vi "ScriptParser.vi"(0 "File Path Control":path, 1 "storage refnum (file) out":refnum<k20>, 2 "ResultaFileName":string, 3 "Array":string[](array[string]), 4 "I":dbl) -> ()   [LabVIEW 2014]
uses:
  <vilib>/Platform/storage/Storage.llb/usiSequenceRepresentation.ctl
  <vilib>/Platform/storage/lvStorage.llb/_queryPropPoly.vi
  <vilib>/Platform/storage/lvStorage.llb/_queryPropString.vi
  <vilib>/Platform/storage/lvStorage.llb/_queryGenericObjects.vi
  <vilib>/Platform/storage/lvStorage.llb/_loadAllDdt.vi
  <vilib>/Platform/storage/lvStorage.llb/xStorage/xStorageSupp/ErrorOut.vi
  <vilib>/Platform/storage/lvStorage.llb/_createOrGetByNameExplicitChildObject.vi
  <vilib>/Platform/storage/Storage.llb/__savePropString.vi
  <vilib>/Platform/storage/lvStorage.llb/__saveFloat64Channel.vi
  <vilib>/Platform/storage/lvStorage.llb/_openStorageWithRootAutoDetect.vi
  <vilib>/Platform/storage/Storage.llb/__savePropTime.vi
  <vilib>/Platform/storage/Storage.llb/Get Object Info.vi
  <vilib>/Platform/storage/Storage.llb/__closeStorageFromObject.vi
  <vilib>/Platform/storage/lvStorage.llb/xStorage/Read Data/Read Data.xnode
  <vilib>/Platform/storage/lvStorage.llb/xStorage/Write Data/Write Data.xnode
  <vilib>/Platform/storage/lvStorage.llb/xStorage/Open Data Storage/Open Data Storage.xnode
  <vilib>/Platform/storage/lvStorage.llb/xStorage/Set Properties/Set Properties.xnode
  <vilib>/Platform/storage/lvStorage.llb/xStorage/Close Data Storage/Close Data Storage.xnode
panel:
  out "Numeric":dbl
  out "storage refnums (channel)":refnum<k20>[](array[refnum])
  out "Default":bool
  # "DEBUG"
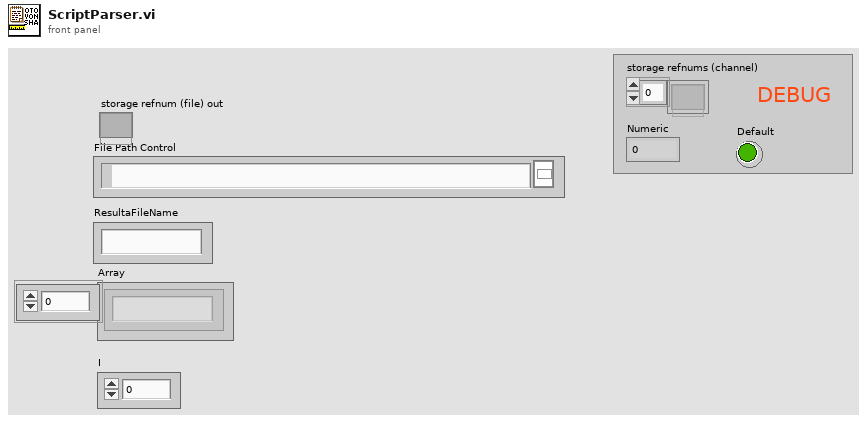
[diagram p1: front panel]
types:
  T1 = enum16{"UPDATE", "READ", "QUERY", "CREATE CHILD", "CREATE", "CONNECT", "DISCONNECT"}
  T2 = enum16{"Append values", "Replace values at index", "Replace all values"}
  T3 = typedef "usiSequenceRepresentation.ctl" = enum16{"explicit", "implicit"}
  T4 = enum16{"open", "open or create", "create or replace", "create", "open (read only)"}
  T5 = typedef "Channel.ctl" = cluster{"AutoLevel":bool, "Thresold":dbl, "Impedance ":dbl, "Voltage Range":dbl, "Active Edge ":i32}
  T6 = typedef "VBreakInitialCond.ctl" = cluster{"Range":dbl, "Ilim":dbl, "Level":dbl, "Channel":i32, "Timed Totalize":dbl}
  T7 = typedef "VBreakStopCondition.ctl" = cluster{"Count Min":dbl, "Count Max":dbl, "Vmax":dbl}
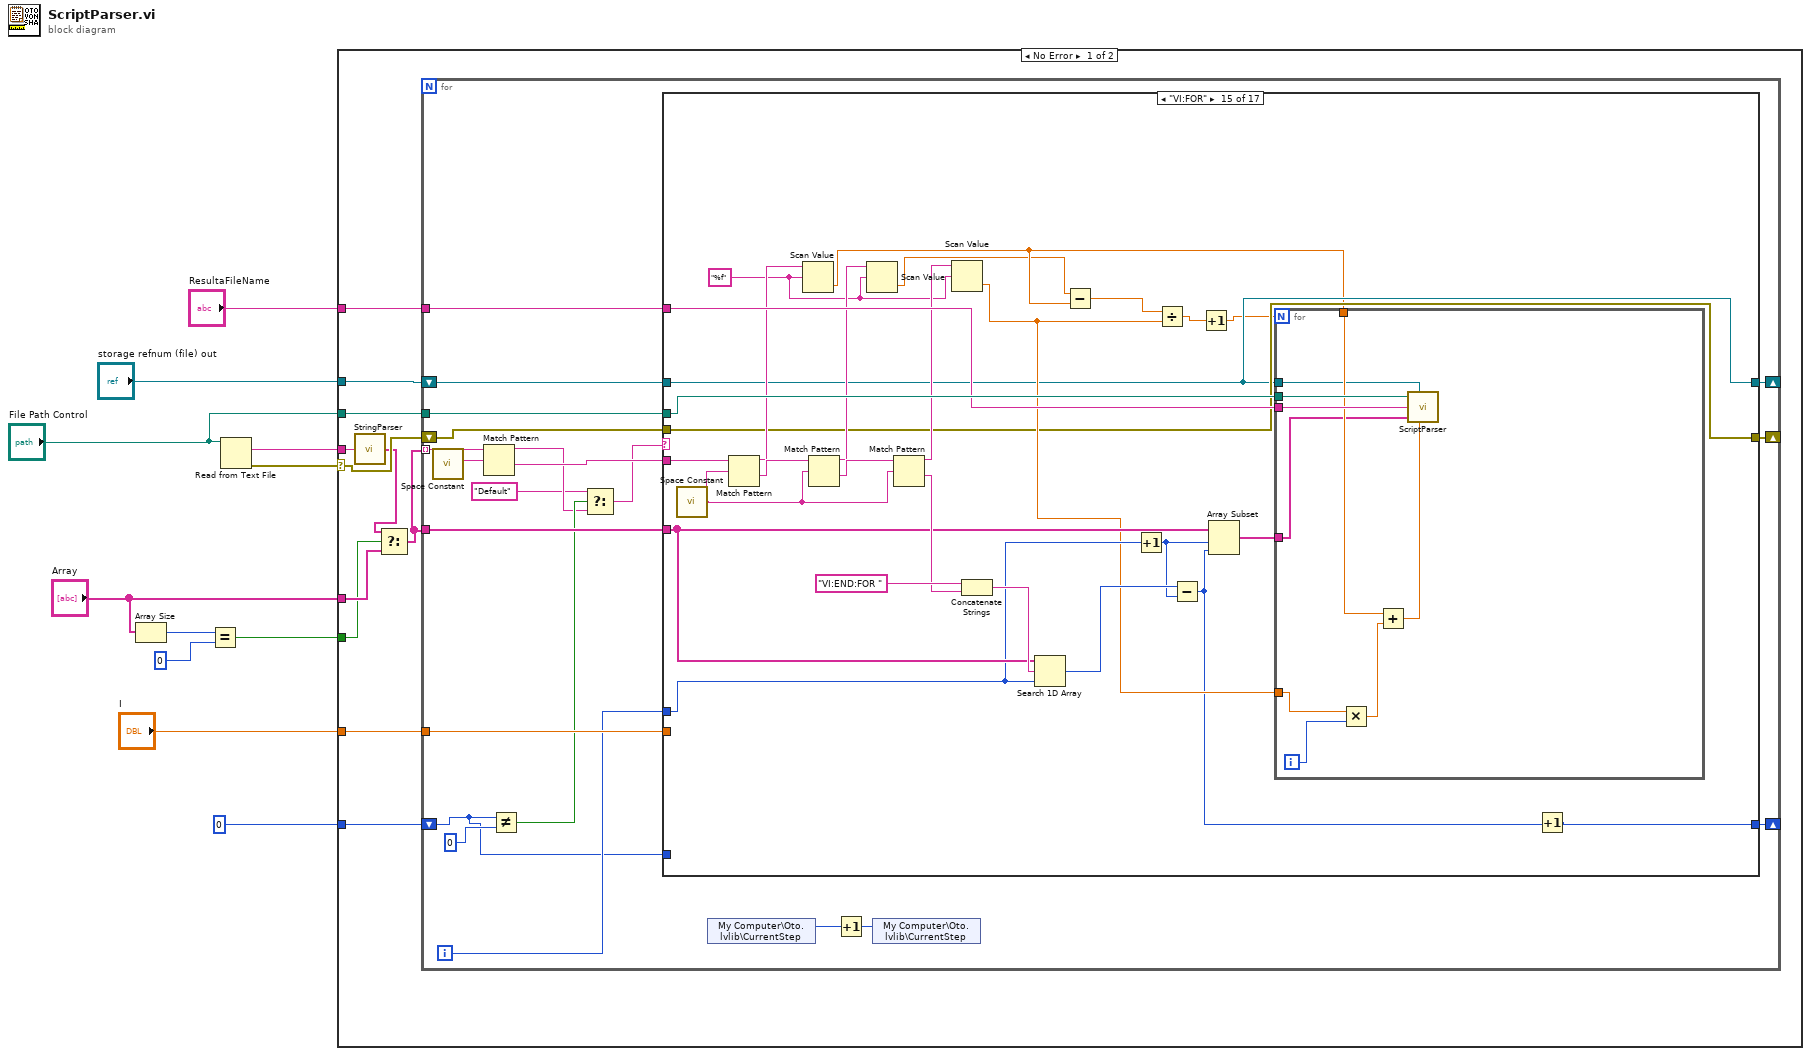
[diagram p0: block diagram]
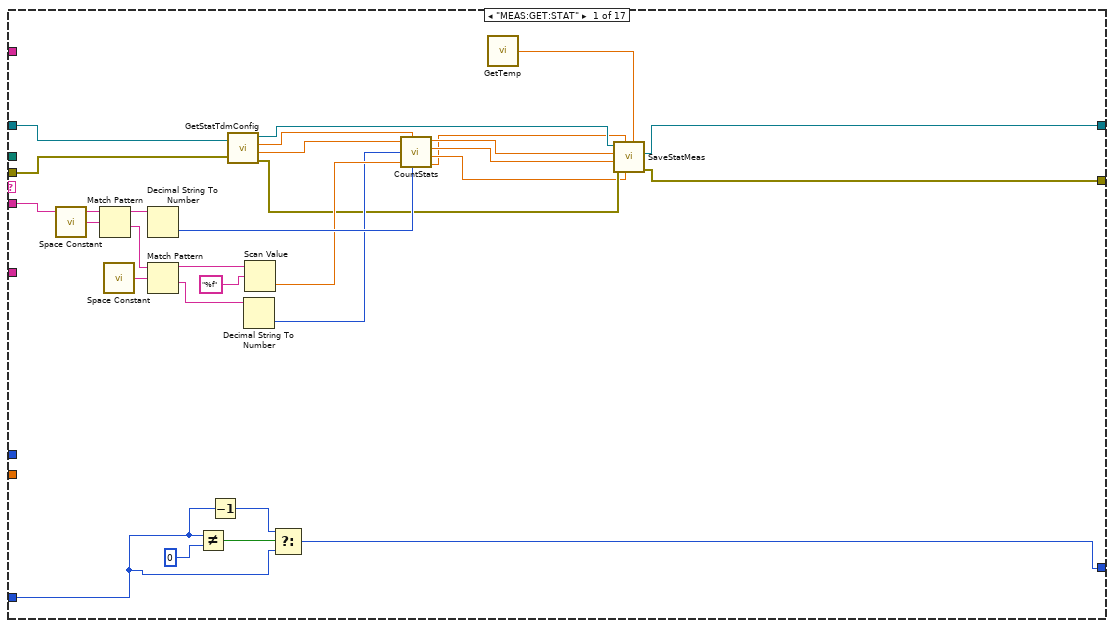
[diagram p2: hidden frame]
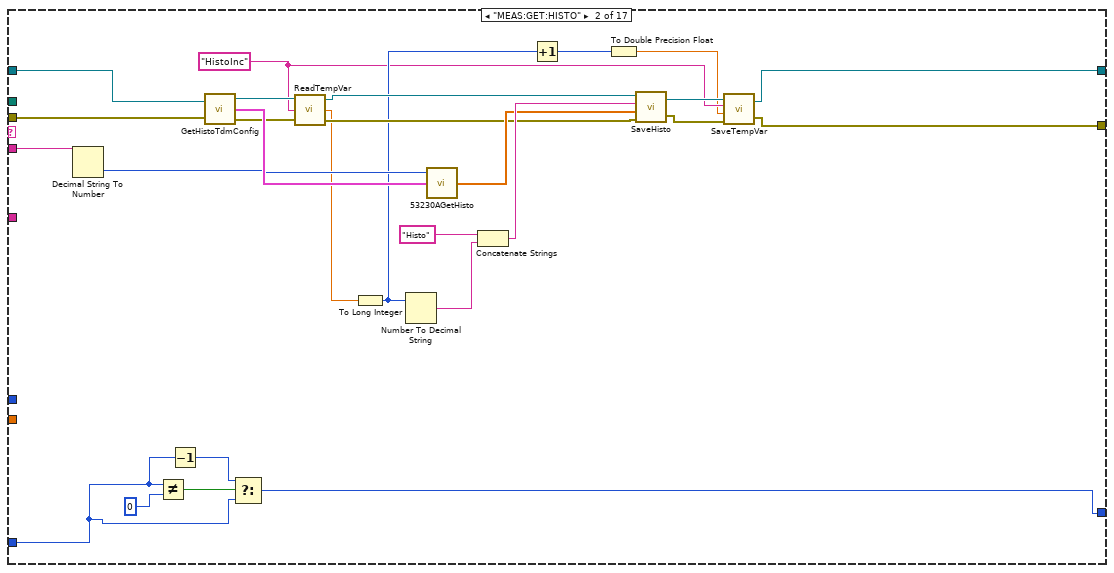
[diagram p3: hidden frame]
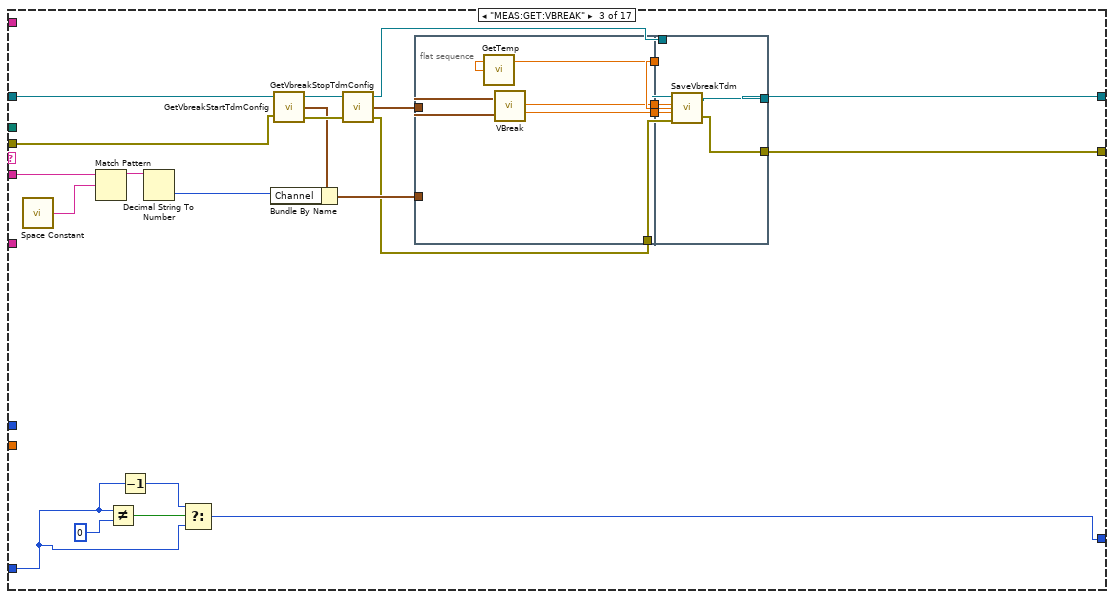
[diagram p4: hidden frame]
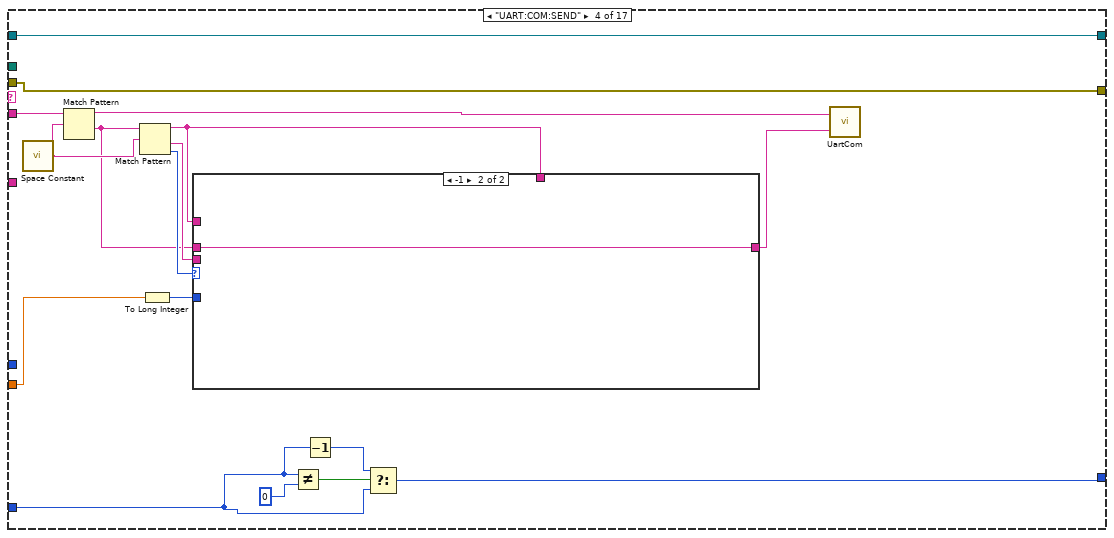
[diagram p5: hidden frame]
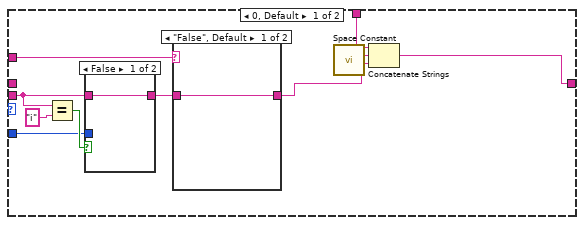
[diagram p6: hidden frame]
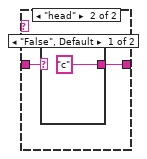
[diagram p7: hidden frame]
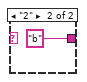
[diagram p8: hidden frame]
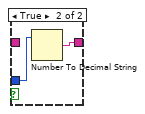
[diagram p9: hidden frame]
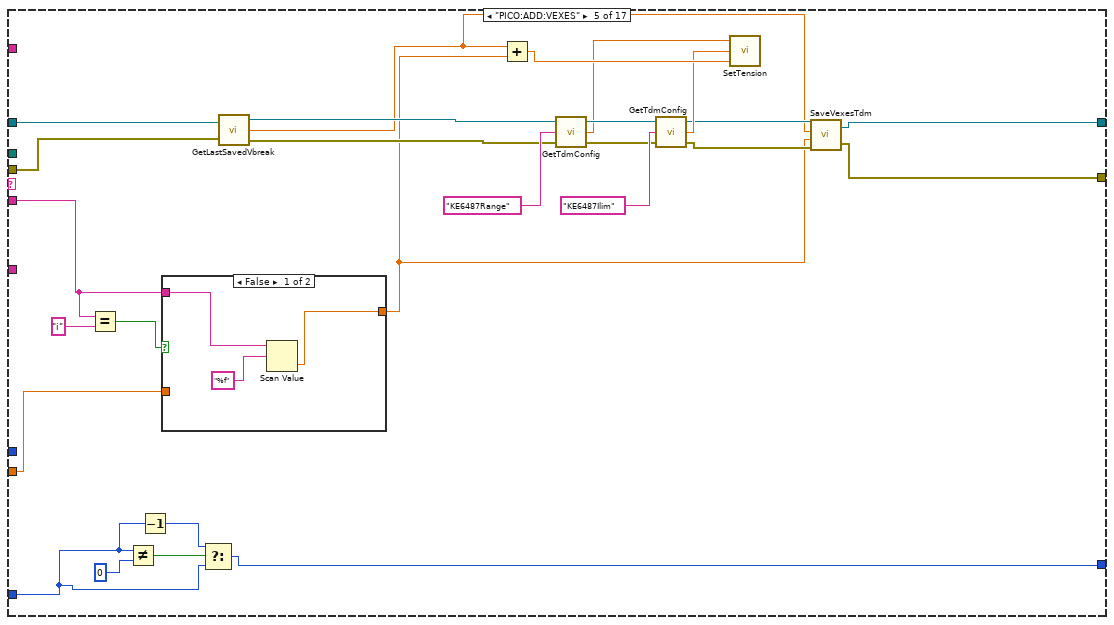
[diagram p10: hidden frame]
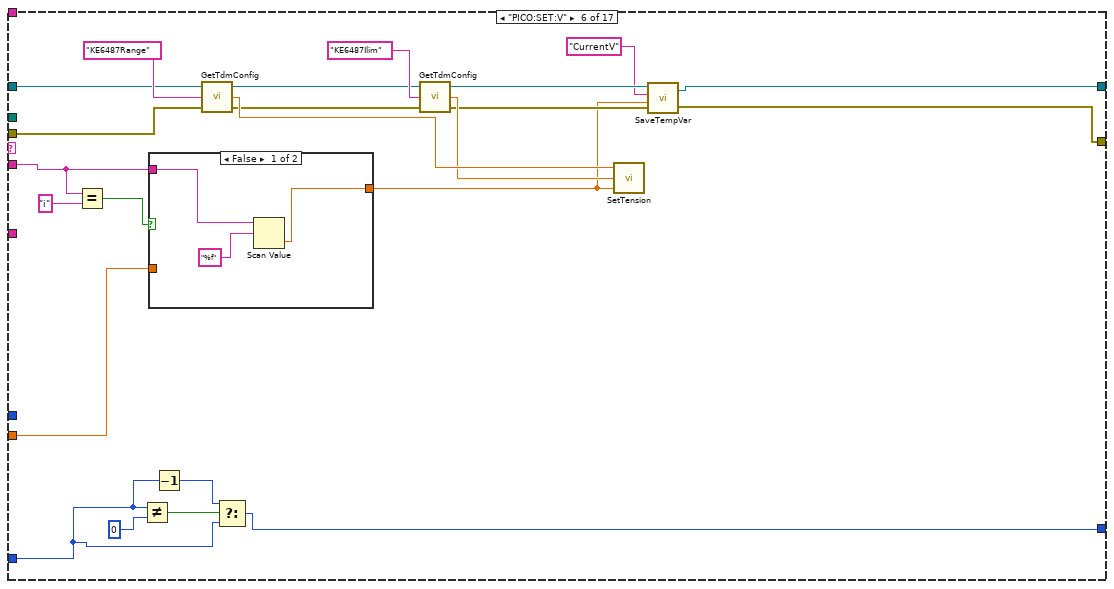
[diagram p12: hidden frame]
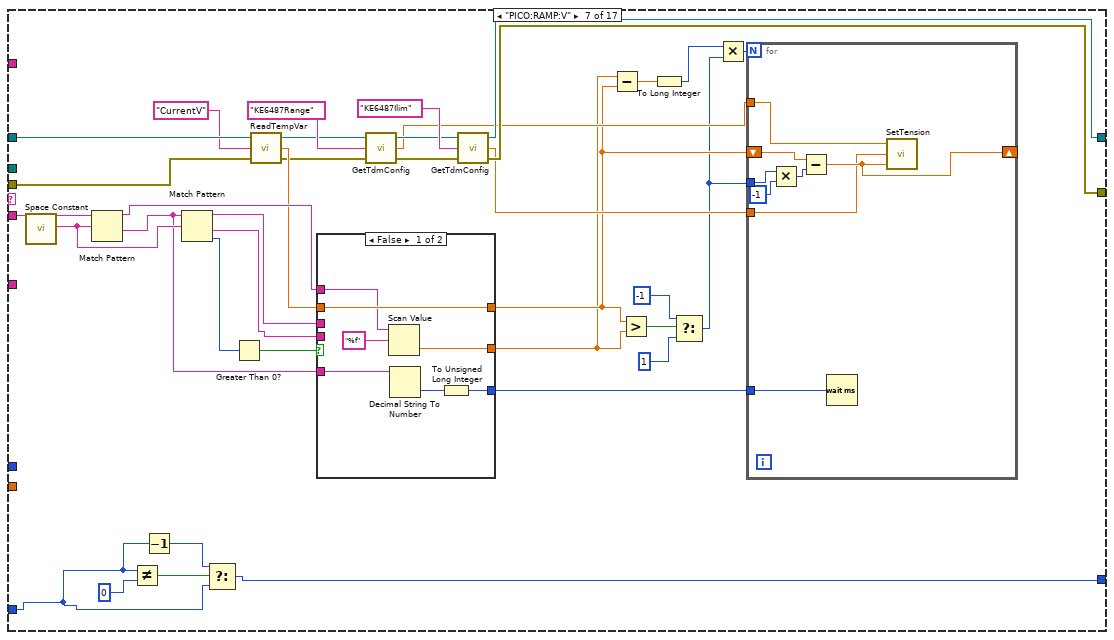
[diagram p14: hidden frame]
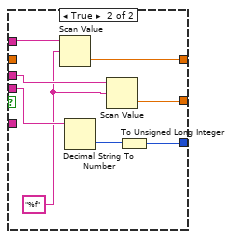
[diagram p15: hidden frame]
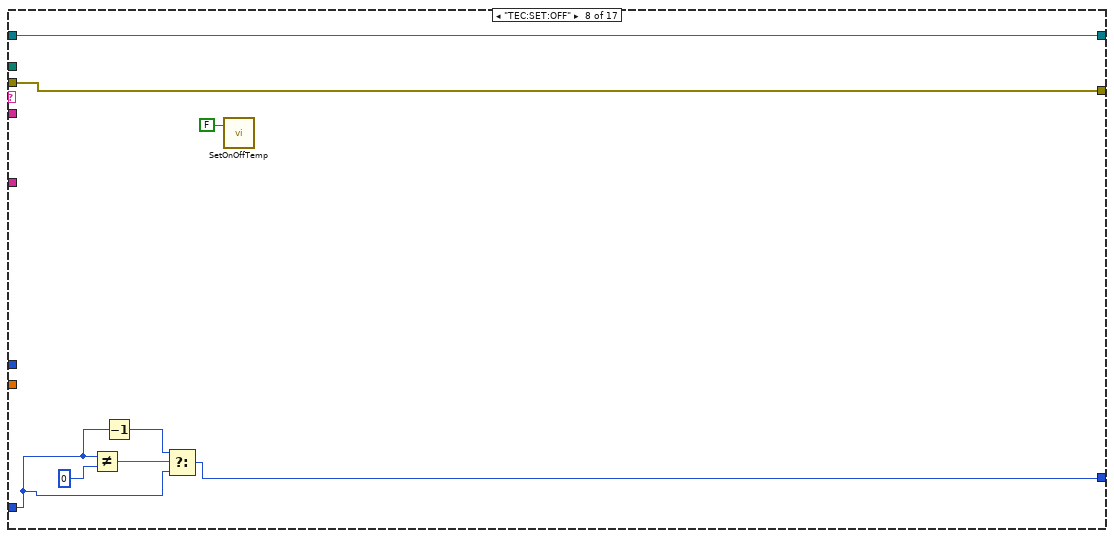
[diagram p16: hidden frame]
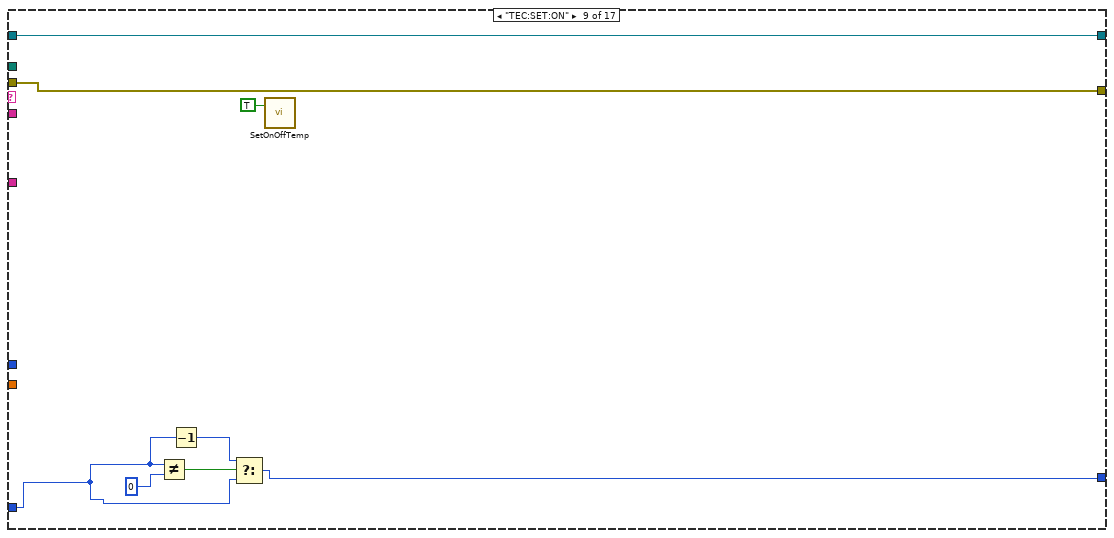
[diagram p17: hidden frame]
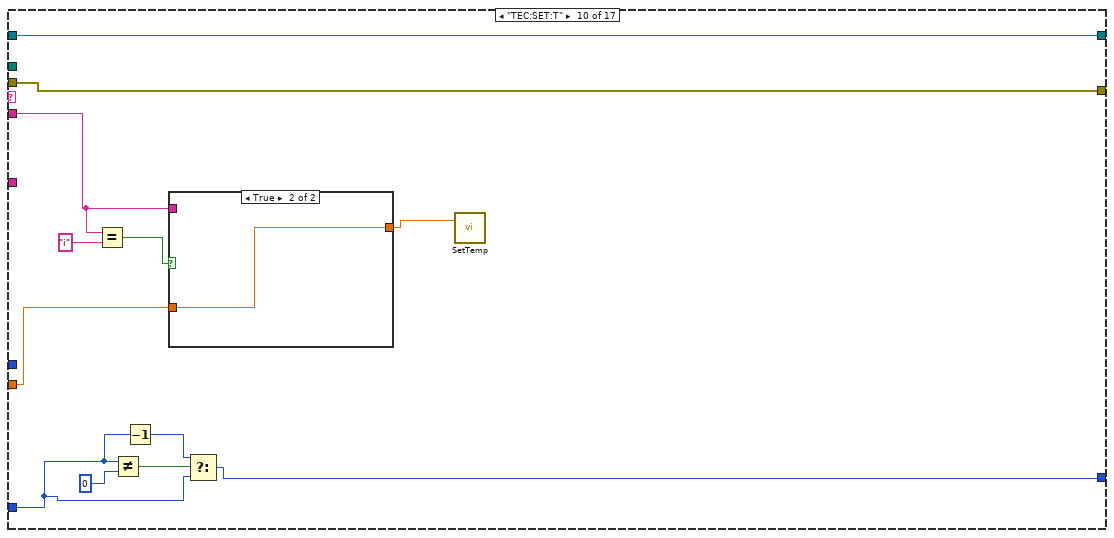
[diagram p18: hidden frame]
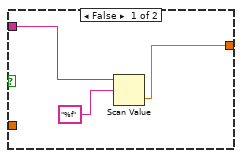
[diagram p19: hidden frame]
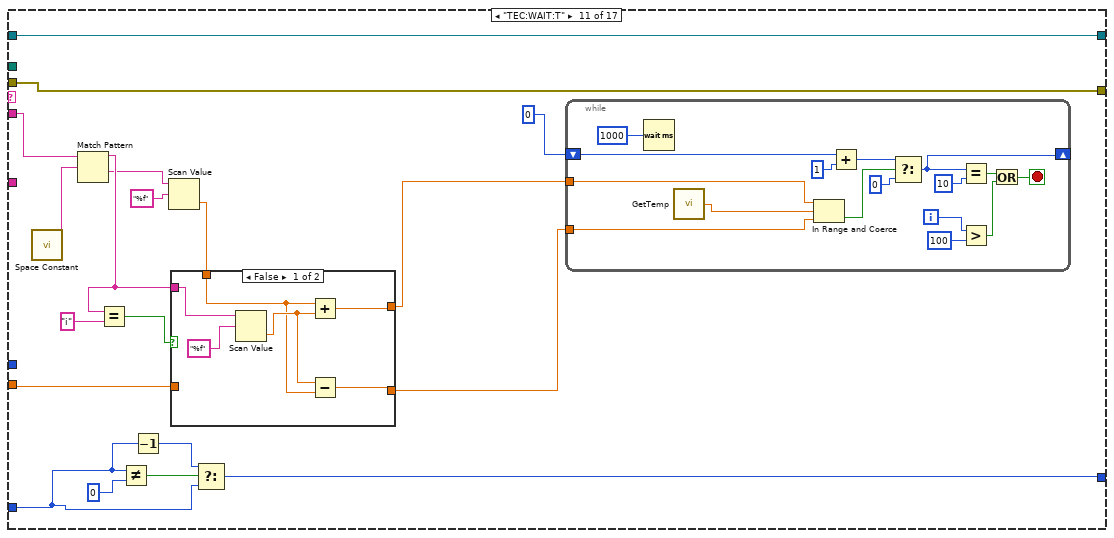
[diagram p20: hidden frame]
diagram:
  n1 = Array Size(array="Array") -> (size(s)=w4:i32)
  n2 = Equal?(x=w4, y=0) -> (x = y?=w2:bool)
  n3 = Read from Text File(file (use dialog)="File Path Control") -> (text=w6:string, error out=w11:errorcluster)  [unwired: 3 in, 2 out]
  n4 = case shown="No Error" w11 {
    selector: w11 -> [w20 _]
    tunnel: w6 -> [w18 _]
    tunnel: "File Path Control" -> [w22 _]
    tunnel: "ResultaFileName" -> [w21 _]
    tunnel: "I" -> [w19 _]
    tunnel: "storage refnum (file) out" -> [w17 _]
    tunnel: "Array" -> [w15 _]
    tunnel: w2 -> [w14 _]
    tunnel: 0 -> [w12 _]
    frame No Error {
      n5 = call "StringParser.vi"("String"=w18) -> ("array"=w16:string[])
      n6 = Select(t=w16, s=w14, f=w15) -> (s? t:f=w13:string[])
      n7 = for {
        tunnel: w13 -> [w42] mode=indexing
        tunnel: w22 -> [w37]
        tunnel: w21 -> [w40]
        shift-right: [w39] -> _
        shift-left: w17 -> [w36]
        shift-right: [w38] -> _
        shift-left: w20 -> [w35]
        tunnel: w19 -> [w34]
        tunnel: w13 -> [w33]
        shift-right: [w26] -> _
        shift-left: w12 -> [w25]
        i -> [w32]
        n8 = call <vilib>:"Space Constant.vi"() -> ("String"=w43:string)
        n9 = Match Pattern(string=w42, regular expression=w43) -> (before substring=w29:string, after substring=w41:string)  [unwired: 1 in, 2 out]
        n10 = Not Equal?(x=w25, y=0) -> (x != y?=w30:bool)
        n11 = Select(t="Default", s=w30, f=w29) -> (s? t:f=w27:string)
        n12 = case shown="\"VI:FOR\"" w27 {
          tunnel: w41 -> [w69 w91 w116 w151 w178 w213 w264 _ _ w310 w326 w377 w414 _ w532 _ _]
          tunnel: w37 -> [_ _ _ _ _ _ _ _ _ _ _ _ _ w469 w521 _ _]
          tunnel: w40 -> [_ _ _ _ _ _ _ _ _ _ _ _ _ w456 w519 _ _]
          tunnel: [w51 w74 w101 w147 w174 w204 w244 w294 w302 w315 w336 w372 w403 w452 w511 w547 w564] -> w39
          tunnel: [w50 w73 w100 w146 w173 w203 w243 w293 w301 w314 w335 w371 w402 w450 w512 w548 w563] -> w38
          tunnel: w36 -> [w72 w98 w122 w147 w196 w219 w263 w294 w302 w315 w336 w373 w404 _ w511 w547 w564]
          tunnel: w35 -> [w71 w97 w121 w146 w195 w218 w262 w293 w301 w314 w335 w370 w401 _ w512 w549 w563]
          tunnel: w34 -> [_ _ _ w140 w177 w212 _ _ _ w311 w327 _ _ _ _ _ _]
          tunnel: w33 -> [_ _ _ _ _ _ _ _ _ _ _ _ _ _ w525 _ _]
          tunnel: w32 -> [_ _ _ _ _ _ _ _ _ _ _ _ _ _ w523 _ _]
          tunnel: [w45 w92 w107 w141 w183 w207 w236 w288 w296 w304 w330 w365 w396 w457 w507 w542 w558] -> w26
          tunnel: w25 -> [w46 w93 w108 w142 w184 w208 w237 w289 w297 w305 w331 w366 w397 w458 _ w543 w559]
          frame "MEAS:GET:STAT" {
            n13 = call <vilib>:"Space Constant.vi"() -> ("String"=w70:string)
            n14 = Match Pattern(string=w69, regular expression=w70) -> (before substring=w66:string, after substring=w63:string)  [unwired: 1 in, 2 out]
            n15 = call <vilib>:"Space Constant.vi"() -> ("String"=w64:string)
            n16 = Decimal String To Number(string=w66) -> (number=w65:i32)  [unwired: 2 in, 1 out]
            n17 = Match Pattern(string=w63, regular expression=w64) -> (before substring=w62:string, after substring=w60:string)  [unwired: 1 in, 2 out]
            n18 = Not Equal?(x=w46, y=0) -> (x != y?=w48:bool)
            n19 = Decrement(x=w46) -> (x-1=w47:i32)
            n20 = call "GetStatTdmConfig.vi"("storage refnum (file)"=w72, "error in"=w71) -> ("storage refnum (file) out"=w57:refnum<k20>, "Impedance"=w68:dbl, "Voltage Range"=w67:dbl, "error out"=w56:errorcluster)
            n21 = Decimal String To Number(string=w60) -> (number=w58:i32)  [unwired: 2 in, 1 out]
            n22 = Scan Value(string=w62, format string="%f") -> (value=w59:dbl)  [unwired: 1 in, 1 out]
            n23 = Select(t=w47, s=w48, f=w46) -> (s? t:f=w45:i32)
            n24 = call "CountStats.vi"("Voltage Range (5V)"=w67, "Impedance (1E+6 Ohm)"=w68, "Channel (Channel1)"=w58, "Totalize Timed (s)"=w59, "Points"=w65) -> ("Moyenne"=w55:dbl, "Ecart type"=w54:dbl, "Min"=w53:dbl, "Max"=w52:dbl)
            n25 = call "GetTemp.vi"() -> ("result"=w44:dbl)
            n26 = call "SaveStatMeas.vi"("Temp"=w44, "Min"=w53, "Max"=w52, "error in"=w56, "Ecart Type"=w54, "Moyenne"=w55, "storage refnum (file)"=w57) -> ("error out"=w50:errorcluster, "storage refnum (file) 2"=w51:refnum<k20>)  [unwired: 2 in]
          }
          frame "MEAS:GET:HISTO" {
            w77 = "HistoInc"
            n27 = Decimal String To Number(string=w91) -> (number=w90:i32)  [unwired: 2 in, 1 out]
            n28 = Not Equal?(x=w93, y=0) -> (x != y?=w95:bool)
            n29 = Decrement(x=w93) -> (x-1=w94:i32)
            n30 = call "GetHistoTdmConfig.vi"("storage refnum (file) out"=w98, "error in"=w97) -> ("storage refnum (file) out 2"=w84:refnum<k20>, "output cluster"=w99:T5, "error out"=w83:errorcluster)
            n31 = Select(t=w94, s=w95, f=w93) -> (s? t:f=w92:i32)
            n32 = call "ReadTempVar.vi"("error in"=w83, "Name"=w77, "storage refnum (file)"=w84) -> ("error out"=w81:errorcluster, "Numeric Indicator"=w80:dbl, "storage refnum (file) out"=w82:refnum<k20>)
            n33 = To Long Integer(number=w80) -> (32bit integer=w78:i32)
            n34 = Number To Decimal String(number=w78) -> (decimal integer string=w79:string)  [unwired: 1 in]
            n35 = call "53230AGetHisto.vi"("Channel2"=w99, "Channel1"=w99, "Numeric Control"=w90) -> ("Measurements"=w87:dbl[])
            n36 = Concatenate Strings("Histo" ("string"), w79) -> (w88:string)
            n37 = Increment(x=w78) -> (x+1=w76:i32)
            n38 = To Double Precision Float(number=w76) -> (double precision float=w75:dbl)
            n39 = call "SaveHisto.vi"("error in"=w81, "Array"=w87, "String"=w88, "storage refnum (file)"=w82) -> ("error out"=w85:errorcluster, "storage refnum (file) out"=w86:refnum<k20>)
            n40 = call "SaveTempVar.vi"("error in"=w85, "Val"=w75, "Name"=w77, "storage refnum (file)"=w86) -> ("error out"=w73:errorcluster, "storage refnum (file) out"=w74:refnum<k20>)
          }
          frame "MEAS:GET:VBREAK" {
            n41 = call <vilib>:"Space Constant.vi"() -> ("String"=w117:string)
            n42 = Match Pattern(string=w116, regular expression=w117) -> (before substring=w115:string)  [unwired: 1 in, 3 out]
            n43 = Not Equal?(x=w108, y=0) -> (x != y?=w110:bool)
            n44 = Decrement(x=w108) -> (x-1=w109:i32)
            n45 = Decimal String To Number(string=w115) -> (number=w113:i32)  [unwired: 2 in, 1 out]
            n46 = Select(t=w109, s=w110, f=w108) -> (s? t:f=w107:i32)
            n47 = call "GetVbreakStartTdmConfig.vi"("storage refnum (file)"=w122, "error in"=w121) -> ("storage refnum (file) out"=w120:refnum<k20>, "output cluster"=w114:T6, "error out"=w119:errorcluster)
            n48 = Bundle By Name(cluster=w114, "Channel"=w113) -> (w112:T6)
            n49 = call "GetVbreakStopTdmConfig.vi"("storage refnum (file)"=w120, "error in"=w119) -> ("storage refnum (file) out"=w103:refnum<k20>, "output cluster"=w118:T7, "error out"=w102:errorcluster)
            n50 = flat-sequence {
              tunnel: w118 -> [w127]
              tunnel: w112 -> [w123]
              tunnel: [w126] -> w106
              tunnel: [w125] -> w105
              tunnel: [w124] -> w104
              tunnel: w106 -> [w133]
              tunnel: w105 -> [w132]
              tunnel: w104 -> [w134]
              tunnel: w103 -> [w130]
              tunnel: w102 -> [w131]
              tunnel: [w129] -> w101
              tunnel: [w128] -> w100
              frame #0 {
                n51 = call "GetTemp.vi"() -> ("result"=w124:dbl)
                n52 = call "VBreak.vi"("Condition d'arret"=w127, "Condition Initial"=w123) -> ("VBreak"=w126:dbl, "Count"=w125:dbl)
              }
              frame #1 {
                n53 = call "SaveVbreakTdm.vi"("storage refnum (file)"=w130, "Vbreak"=w133, "Count"=w132, "error in"=w131, "Temp"=w134) -> ("storage refnum (file) 2"=w129:refnum<k20>, "error out"=w128:errorcluster)
              }
            }
          }
          frame "UART:COM:SEND" {
            n54 = call <vilib>:"Space Constant.vi"() -> ("String"=w149:string)
            n55 = Match Pattern(string=w151, regular expression=w149) -> (before substring=w150:string, after substring=w137:string)  [unwired: 1 in, 2 out]
            n56 = Match Pattern(string=w137, regular expression=w149) -> (before substring=w136:string, after substring=w148:string, offset past match=w138:i32)  [unwired: 1 in, 1 out]
            n57 = To Long Integer(number=w140) -> (32bit integer=w139:i32)
            n58 = case shown="-1" w138 {
              tunnel: w148 -> [w159 _]
              tunnel: [w153 w170] -> w135
              tunnel: w136 -> [w157 _]
              tunnel: w139 -> [w156 _]
              tunnel: w137 -> [_ w170]
              tunnel: w136 -> [w152 _]
              frame 0, Default {
                n59 = Equal?(x=w159, y="i") -> (x = y?=w160:bool)
                n60 = case shown="False" w160 {
                  tunnel: w159 -> [w167 _]
                  tunnel: w156 -> [_ w169]
                  tunnel: [w167 w168] -> w158
                  frame False {
                  }
                  frame True {
                    n61 = Number To Decimal String(number=w169) -> (decimal integer string=w168:string)  [unwired: 1 in]
                  }
                }
                n62 = case shown="\"False\", Default" w157 {
                  tunnel: w158 -> [w162 w164]
                  tunnel: [w162 w163] -> w154
                  frame "False", Default {
                  }
                  frame "head" {
                    n63 = case shown="\"False\", Default" w164 {
                      tunnel: ["c" "b"] -> w163
                      frame "False", Default {
                      }
                      frame "2" {
                      }
                    }
                  }
                }
                n64 = call <vilib>:"Space Constant.vi"() -> ("String"=w155:string)
                n65 = Concatenate Strings(w152, w155, w154) -> (w153:string)
              }
              frame -1 {
              }
            }
            n66 = Not Equal?(x=w142, y=0) -> (x != y?=w144:bool)
            n67 = Decrement(x=w142) -> (x-1=w143:i32)
            n68 = Select(t=w143, s=w144, f=w142) -> (s? t:f=w141:i32)
            n69 = call "UartCom.vi"("String"=w135, "VISA resource name"=w150) -> ()  [unwired: 1 out]
          }
          frame "PICO:ADD:VEXES" {
            n70 = Equal?(x=w178, y="i") -> (x = y?=w179:bool)
            n71 = Not Equal?(x=w184, y=0) -> (x != y?=w186:bool)
            n72 = Decrement(x=w184) -> (x-1=w185:i32)
            n73 = case shown="False" w179 {
              tunnel: w178 -> [w198 _]
              tunnel: [w197 w200] -> w171
              tunnel: w177 -> [_ w200]
              frame False {
                n74 = Scan Value(string=w198, format string="%f") -> (value=w197:dbl)  [unwired: 1 in, 1 out]
              }
              frame True {
              }
            }
            n75 = Select(t=w185, s=w186, f=w184) -> (s? t:f=w183:i32)
            n76 = call "GetLastSavedVbreak.vi"("storage refnum (file)"=w196, "error in"=w195) -> ("storage refnum (file) out"=w182:refnum<k20>, "VBreak"=w172:dbl, "error out"=w181:errorcluster)
            n77 = Add(x=w172, y=w171) -> (x+y=w190:dbl)
            n78 = call "GetTdmConfig.vi"("error in 2"=w181, "String"="KE6487Range", "storage refnum (file)"=w182) -> ("error in"=w191:errorcluster, "Numeric"=w189:dbl, "storage refnum (file) out"=w192:refnum<k20>)
            n79 = call "GetTdmConfig.vi"("error in 2"=w191, "String"="KE6487Ilim", "storage refnum (file)"=w192) -> ("error in"=w175:errorcluster, "Numeric"=w188:dbl, "storage refnum (file) out"=w176:refnum<k20>)
            n80 = call "SetTension.vi"("level"=w190, "compliance limit"=w188, "range"=w189) -> ()
            n81 = call "SaveVexesTdm.vi"("error in"=w175, "VExes"=w171, "Vbreak"=w172, "storage refnum (file)"=w176) -> ("error out"=w173:errorcluster, "storage refnum (file) 3"=w174:refnum<k20>)
          }
          frame "PICO:SET:V" {
            n82 = Equal?(x=w213, y="i") -> (x = y?=w214:bool)
            n83 = Not Equal?(x=w208, y=0) -> (x != y?=w210:bool)
            n84 = case shown="False" w214 {
              tunnel: w213 -> [w225 _]
              tunnel: [w224 w227] -> w202
              tunnel: w212 -> [_ w227]
              frame False {
                n85 = Scan Value(string=w225, format string="%f") -> (value=w224:dbl)  [unwired: 1 in, 1 out]
              }
              frame True {
              }
            }
            n86 = Decrement(x=w208) -> (x-1=w209:i32)
            n87 = call "GetTdmConfig.vi"("error in 2"=w218, "String"="KE6487Range", "storage refnum (file)"=w219) -> ("error in"=w216:errorcluster, "Numeric"=w223:dbl, "storage refnum (file) out"=w217:refnum<k20>)
            n88 = Select(t=w209, s=w210, f=w208) -> (s? t:f=w207:i32)
            n89 = call "GetTdmConfig.vi"("error in 2"=w216, "String"="KE6487Ilim", "storage refnum (file)"=w217) -> ("error in"=w205:errorcluster, "Numeric"=w222:dbl, "storage refnum (file) out"=w206:refnum<k20>)
            n90 = call "SetTension.vi"("level"=w202, "compliance limit"=w222, "range"=w223) -> ()
            n91 = call "SaveTempVar.vi"("error in"=w205, "Val"=w202, "Name"="CurrentV", "storage refnum (file)"=w206) -> ("error out"=w203:errorcluster, "storage refnum (file) out"=w204:refnum<k20>)
          }
          frame "PICO:RAMP:V" {
            n92 = call <vilib>:"Space Constant.vi"() -> ("String"=w260:string)
            n93 = Match Pattern(string=w264, regular expression=w260) -> (before substring=w257:string, after substring=w253:string)  [unwired: 1 in, 2 out]
            n94 = Not Equal?(x=w237, y=0) -> (x != y?=w239:bool)
            n95 = Decrement(x=w237) -> (x-1=w238:i32)
            n96 = Match Pattern(string=w253, regular expression=w260) -> (before substring=w255:string, after substring=w254:string, offset past match=w259:i32)  [unwired: 1 in, 1 out]
            n97 = Select(t=w238, s=w239, f=w237) -> (s? t:f=w236:i32)
            n98 = Greater Than 0?(x=w259) -> (x > 0?=w258:bool)
            n99 = call "ReadTempVar.vi"("error in"=w262, "Name"="CurrentV", "storage refnum (file)"=w263) -> ("error out"=w246:errorcluster, "Numeric Indicator"=w256:dbl, "storage refnum (file) out"=w245:refnum<k20>)
            n100 = case shown="False" w258 {
              tunnel: w257 -> [w278 w287]
              tunnel: [w279 w286] -> w235
              tunnel: w256 -> [w279 _]
              tunnel: w255 -> [_ w282]
              tunnel: w254 -> [_ w285]
              tunnel: w253 -> [w276 _]
              tunnel: [w277 w280] -> w234
              tunnel: [w274 w283] -> w252
              frame False {
                n101 = Scan Value(string=w278, format string="%f") -> (value=w277:dbl)  [unwired: 1 in, 1 out]
                n102 = Decimal String To Number(string=w276) -> (number=w275:i32)  [unwired: 2 in, 1 out]
                n103 = To Unsigned Long Integer(number=w275) -> (unsigned 32bit integer=w274:u32)
              }
              frame True {
                w281 = "%f" ("format string")
                n104 = Scan Value(string=w287, format string=w281) -> (value=w286:dbl)  [unwired: 1 in, 1 out]
                n105 = Decimal String To Number(string=w285) -> (number=w284:i32)  [unwired: 2 in, 1 out]
                n106 = Scan Value(string=w282, format string=w281) -> (value=w280:dbl)  [unwired: 1 in, 1 out]
                n107 = To Unsigned Long Integer(number=w284) -> (unsigned 32bit integer=w283:u32)
              }
            }
            n108 = call "GetTdmConfig.vi"("error in 2"=w246, "String"="KE6487Range", "storage refnum (file)"=w245) -> ("error in"=w247:errorcluster, "Numeric"=w242:dbl, "storage refnum (file) out"=w248:refnum<k20>)
            n109 = call "GetTdmConfig.vi"("error in 2"=w247, "String"="KE6487Ilim", "storage refnum (file)"=w248) -> ("error in"=w243:errorcluster, "Numeric"=w241:dbl, "storage refnum (file) out"=w244:refnum<k20>)
            n110 = Subtract(x=w234, y=w235) -> (x-y=w251:dbl)
            n111 = Greater?(x=w235, y=w234) -> (0:w233:bool)
            n112 = To Long Integer(number=w251) -> (32bit integer=w230:i32)
            n113 = Select(t=-1, s=w233, f=1) -> (s? t:f=w228:i32)
            n114 = Multiply(x=w230, y=w228) -> (x*y=w229:i32)
            n115 = for {
              N: w229 -> [_]
              tunnel: w252 -> [w272]
              shift-right: [w270] -> _
              shift-left: w235 -> [w271]
              tunnel: w242 -> [w269]
              tunnel: w241 -> [w268]
              tunnel: w228 -> [w266]
              n116 = Multiply(x=w266, y=-1) -> (x*y=w267:i32)
              n117 = Subtract(x=w271, y=w267) -> (x-y=w270:dbl)
              n118 = Wait (ms)(milliseconds to wait=w272) -> ()  [unwired: 1 out]
              n119 = call "SetTension.vi"("level"=w270, "compliance limit"=w268, "range"=w269) -> ()
            }
          }
          frame "TEC:SET:OFF" {
            n120 = Not Equal?(x=w289, y=0) -> (x != y?=w291:bool)
            n121 = Decrement(x=w289) -> (x-1=w290:i32)
            n122 = Select(t=w290, s=w291, f=w289) -> (s? t:f=w288:i32)
            n123 = call "SetOnOffTemp.vi"("Boolean"=FALSE) -> ()  [unwired: 1 in, 1 out]
          }
          frame "TEC:SET:ON" {
            n124 = Not Equal?(x=w297, y=0) -> (x != y?=w299:bool)
            n125 = Decrement(x=w297) -> (x-1=w298:i32)
            n126 = Select(t=w298, s=w299, f=w297) -> (s? t:f=w296:i32)
            n127 = call "SetOnOffTemp.vi"("Boolean"=TRUE) -> ()  [unwired: 1 in, 1 out]
          }
          frame "TEC:SET:T" {
            n128 = Equal?(x=w310, y="i") -> (x = y?=w312:bool)
            n129 = Not Equal?(x=w305, y=0) -> (x != y?=w307:bool)
            n130 = Decrement(x=w305) -> (x-1=w306:i32)
            n131 = case shown="True" w312 {
              tunnel: w310 -> [w317 _]
              tunnel: [w316 w319] -> w309
              tunnel: w311 -> [_ w319]
              frame False {
                n132 = Scan Value(string=w317, format string="%f") -> (value=w316:dbl)  [unwired: 1 in, 1 out]
              }
              frame True {
              }
            }
            n133 = Select(t=w306, s=w307, f=w305) -> (s? t:f=w304:i32)
            n134 = call "SetTemp.vi"("Numeric Control"=w309) -> ()  [unwired: 1 in, 1 out]
          }
          frame "TEC:WAIT:T" {
            n135 = call <vilib>:"Space Constant.vi"() -> ("String"=w338:string)
            n136 = Match Pattern(string=w326, regular expression=w338) -> (before substring=w325:string, after substring=w323:string)  [unwired: 1 in, 2 out]
            n137 = Equal?(x=w325, y="i") -> (x = y?=w328:bool)
            n138 = Not Equal?(x=w331, y=0) -> (x != y?=w333:bool)
            n139 = Decrement(x=w331) -> (x-1=w332:i32)
            n140 = Scan Value(string=w323, format string="%f") -> (value=w322:dbl)  [unwired: 1 in, 1 out]
            n141 = case shown="False" w328 {
              tunnel: w325 -> [w343 _]
              tunnel: [w339 w346] -> w321
              tunnel: w327 -> [_ w348]
              tunnel: w322 -> [w341 w347]
              tunnel: [w340 w345] -> w320
              frame False {
                n142 = Scan Value(string=w343, format string="%f") -> (value=w342:dbl)  [unwired: 1 in, 1 out]
                n143 = Add(x=w341, y=w342) -> (x+y=w339:dbl)
                n144 = Subtract(x=w342, y=w341) -> (x-y=w340:dbl)
              }
              frame True {
                n145 = Add(x=w348, y=w347) -> (x+y=w346:dbl)
                n146 = Subtract(x=w348, y=w347) -> (x-y=w345:dbl)
              }
            }
            n147 = Select(t=w332, s=w333, f=w331) -> (s? t:f=w330:i32)
            n148 = while {
              tunnel: w321 -> [w363]
              tunnel: w320 -> [w364]
              shift-right: [w357] -> _
              shift-left: 0 -> [w360]
              i -> [w353]
              stop <- w354 stop-if-true
              n149 = Wait (ms)(milliseconds to wait=u32 1000) -> ()  [unwired: 1 out]
              n150 = call "GetTemp.vi"() -> ("result"=w349:dbl)
              n151 = In Range and Coerce(upper limit=w363, x=w349, lower limit=w364) -> (In Range?=w362:bool)  [unwired: 1 out]
              n152 = Add(x=w360, y=1) -> (x+y=w358:i32)
              n153 = Select(t=w358, s=w362, f=0) -> (s? t:f=w357:i32)
              n154 = Equal?(x=w357, y=10) -> (x = y?=w355:bool)
              n155 = Greater?(x=w353, y=100) -> (0:w351:bool)
              n156 = Or(x=w355, y=w351) -> (x .or. y?=w354:bool)
            }
          }
          frame "VI:CONFIG:GET" {
            n157 = Not Equal?(x=w366, y=0) -> (x != y?=w368:bool)
            n158 = Decrement(x=w366) -> (x-1=w367:i32)
            n159 = Select(t=w367, s=w368, f=w366) -> (s? t:f=w365:i32)
            n160 = Wait (ms)(milliseconds to wait=u32 2000) -> ()  [unwired: 1 out]
            n161 = xnode "Read Data\n[Channel]"("Name"=w377, "storage refnum (file)"=w373, "error in"=w370) -> ("storage refnums (channel)"=→"storage refnums (channel)":refnum<k20>[], "Signal"=→"Numeric":dynamicdata, "storage refnum (file) out"=w372:refnum<k20>, "error out"=w371:errorcluster)  [unwired: 3 in]
          }
          frame "VI:CONFIG:SET" {
            n162 = call <vilib>:"Space Constant.vi"() -> ("String"=w413:string)
            n163 = Not Equal?(x=w397, y=0) -> (x != y?=w399:bool)
            n164 = Decrement(x=w397) -> (x-1=w398:i32)
            n165 = Match Pattern(string=w414, regular expression=w413) -> (before substring=w412:string, after substring=w411:string)  [unwired: 1 in, 2 out]
            n166 = Select(t=w398, s=w399, f=w397) -> (s? t:f=w396:i32)
            n167 = Scan Value(string=w411, format string="%f") -> (value=w409:dbl)  [unwired: 1 in, 1 out]
            n168 = xnode "Write Data\n[Channel group]"("Name"="Configs", "storage refnum (file)"=w404, "error in"=w401) -> ("storage refnum (file) out"=w403:refnum<k20>, "error out"=w408:errorcluster, "storage refnum (channel group)"=w406:refnum<k20>)
            n169 = xnode "Write Data\n[Channel]"("Name"=w412, "Signal"=w409, "storage refnum (channel group)"=w406, "error in"=w408, "append / replace (append data values)"=T2."Replace all values") -> ("error out"=w402:errorcluster)  [unwired: 1 in, 2 out]
          }
          frame "VI:INIT" {
            n170 = Not Equal?(x=w458, y=0) -> (x != y?=w460:bool)
            n171 = Decrement(x=w458) -> (x-1=w459:i32)
            n172 = Strip Path(path=w469) -> (stripped path=w470:path)  [unwired: 1 out]
            n173 = Concatenate Strings(w456, ".tdm" ("string")) -> (w454:string)
            n174 = Select(t=w459, s=w460, f=w458) -> (s? t:f=w457:i32)
            n175 = Build Path(base path=w470, name or relative path=w454) -> (appended path=w468:path)
            n176 = xnode "Open Data Storage\n[TDM]"("file path"=w468, "function (open:0)"=T4."open or create") -> ("storage refnum (file)"=w466:refnum<k20>, "error out"=w465:errorcluster)  [unwired: 3 in, 1 out]
            n177 = Get Date/Time In Seconds() -> (seconds since 1Jan1904=w463:timestamp)
            n178 = xnode "Set Properties\n[File]"("Name"="Oto Von Schaft Measurment", "Time stamp"=w463, "Author"="Oto Von Schaft", "storage refnum (file)"=w466, "error in"=w465) -> ("storage refnum (file) out"=w453:refnum<k20>, "error out"=w451:errorcluster)  [unwired: 2 in]
            n179 = call "SaveTempVar.vi"("error in"=w451, "Val"=1.0, "Name"="HistoInc", "storage refnum (file)"=w453) -> ("error out"=w450:errorcluster, "storage refnum (file) out"=w452:refnum<k20>)
          }
          frame "VI:FOR" {
            w515 = "%f" ("format string")
            n180 = call <vilib>:"Space Constant.vi"() -> ("String"=w529:string)
            n181 = Match Pattern(string=w532, regular expression=w529) -> (before substring=w518:string, after substring=w531:string)  [unwired: 1 in, 2 out]
            n182 = Scan Value(string=w518, format string=w515) -> (value=w510:dbl)  [unwired: 1 in, 1 out]
            n183 = Match Pattern(string=w531, regular expression=w529) -> (before substring=w517:string, after substring=w530:string)  [unwired: 1 in, 2 out]
            n184 = Scan Value(string=w517, format string=w515) -> (value=w509:dbl)  [unwired: 1 in, 1 out]
            n185 = Match Pattern(string=w530, regular expression=w529) -> (before substring=w516:string, after substring=w527:string)  [unwired: 1 in, 2 out]
            n186 = Scan Value(string=w516, format string=w515) -> (value=w513:dbl)  [unwired: 1 in, 1 out]
            n187 = Concatenate Strings("VI:END:FOR " ("string"), w527) -> (w526:string)
            n188 = Search 1D Array(1D array=w525, element=w526, start index (0)=w523) -> (index of element=w524:i32)
            n189 = Subtract(x=w509, y=w510) -> (x-y=w514:dbl)
            n190 = Increment(x=w523) -> (x+1=w522:i32)
            n191 = Divide(x=w514, y=w513) -> (x/y=w506:dbl)
            n192 = Subtract(x=w524, y=w522) -> (x-y=w508:i32)
            n193 = Increment(x=w506) -> (x+1=w505:dbl)
            n194 = Array Subset(array=w525, index=w522, length=w508) -> (w520:string[])
            n195 = for {
              N: w505 -> [_]
              tunnel: w521 -> [w541]
              tunnel: w511 -> [w535]
              tunnel: w520 -> [w533]
              tunnel: w519 -> [w540]
              tunnel: w510 -> [w539]
              tunnel: w513 -> [w538]
              i -> [w534]
              n196 = Multiply(x=w538, y=w534) -> (x*y=w537:dbl)
              n197 = Add(x=w539, y=w537) -> (x+y=w536:dbl)
              n198 = call "ScriptParser.vi"("File Path Control"=w541, "storage refnum (file) out"=w535, "ResultaFileName"=w540, "Array"=w533, "I"=w536) -> ()  [unwired: 1 in]
            }
            n199 = Increment(x=w508) -> (x+1=w507:i32)
          }
          frame "VI:END" {
            n200 = Not Equal?(x=w543, y=0) -> (x != y?=w545:bool)
            n201 = Decrement(x=w543) -> (x-1=w544:i32)
            n202 = Select(t=w544, s=w545, f=w543) -> (s? t:f=w542:i32)
            n203 = xnode "Close Data Storage\n"("storage refnum (file)"=w547, "error in (no error)"=w549) -> ("error out"=w548:errorcluster)  [unwired: 1 out]
          }
          frame Default {
            n204 = Not Equal?(x=w559, y=0) -> (x != y?=w561:bool)
            n205 = Decrement(x=w559) -> (x-1=w560:i32)
            n206 = Select(t=w560, s=w561, f=w559) -> (s? t:f=w558:i32)
            n207 = flat-sequence {
              frame #0 {
                "Default" <- TRUE ("PicoSetV")
              }
              frame #1 {
                n208 = Wait (ms)(milliseconds to wait=u32 1000) -> ()  [unwired: 1 out]
              }
              frame #2 {
                n209 = local write "Default"(FALSE ("PicoSetV")) -> ()
              }
            }
          }
        }
        n210 = shared-variable "My Computer\\Oto.lvlib\\CurrentStep"() -> (w24:i32)  [unwired: 1 in, 1 out]
        n211 = Increment(x=w24) -> (x+1=w23:i32)
        n212 = shared-variable "My Computer\\Oto.lvlib\\CurrentStep"(w23) -> ()  [unwired: 1 in, 1 out]
      }
    }
    frame Error {
    }
  }
